vi "SphereSecP(t).vi"(6 "strip (cm)":cluster{"radius":dbl, "h":dbl, "w":dbl}={"radius"=10.0, "h"=5.0, "w"=4.0} {"radius" format="%.2f"; "w" format="%.2f"; "h" format="%.2f"}, 7 "Cluster":T1={"r"=0.0, "d"=0.0, "c (cm/s)"=150000.0, "waveform samp rate s"=1500.0, "In focal Zone?"=FALSE} {"r" format="%.2f"; "d" format="%.2f"; "waveform samp rate s" format="%.2e"; "c (cm/s)" format="%.2f"}, 8 "d (depth of curvature)":dbl format="%.2f", 9 "Drive signal":dbl[](array[numeric])=[-0.5634920634920635, -0.6825396825396826, -0.8015873015873016, -0.9920634920634921, -1.1507936507936507, -1.3888888888888888, -1.992063492063492, -4.2063492063492065, -5.888888888888889, 13.023809523809524, 61.32539682539682, 92.83333333333333, 75.10317460317461, 18.126984126984127, -54.93650793650794, -109.60317460317461, -104.22222222222223, 18.134920634920636, 83.33333333333333, 27.27777777777778, -42.19047619047619, -45.63492063492063, 10.15079365079365, 49.05555555555556, 28.19047619047619, -5.658730158730159, -15.261904761904763, -4.4603174603174605, 7.984126984126984, 10.682539682539682, 5.809523809523809, -0.03968253968253968, -2.515873015873016, -1.4841269841269842, 1.0396825396825398, 2.0555555555555554, 0.9523809523809523, -0.6031746031746031, -1.007936507936508, -0.3968253968253968, 0.14285714285714285] format="%.2f", 10 "edge points":dbl[][](array[numeric]) format="%.2f", 11 "P (cm)":cluster{"x":dbl, "y":dbl, "z":dbl}={"x"=-4.0, "y"=0.0, "z"=4.0} {"x" format="%.2f"; "z" format="%.2f"; "y" format="%.2f"}) -> (2 "Pressure Wave":dbl[](graph), 3 "min time shift":dbl format="%.2f")   [LabVIEW 2022 SP3]
uses:
  <vilib>/Analysis/2dsp.llb/1D Convolution (DBL).vi
  <vilib>/Analysis/baseanly.llb/A x Vector.vi
  <vilib>/Analysis/2dsp.llb/Derivative x(t).vi
  <vilib>/Analysis/NI_AALPro.lvlib
  <vilib>/Analysis/NI_AALBase.lvlib
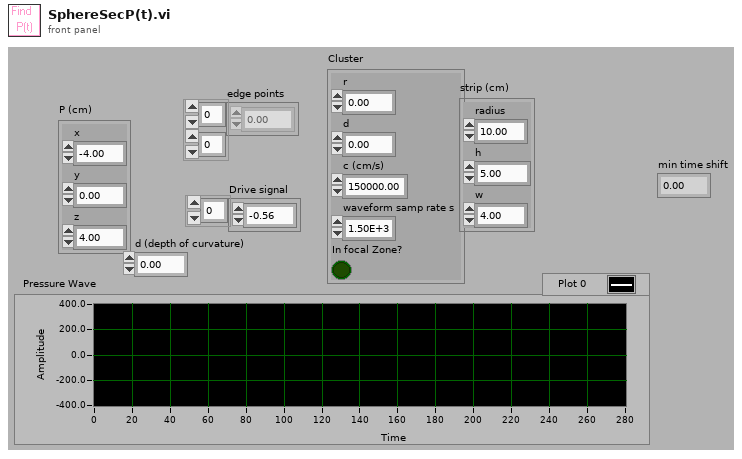
[diagram p1: front panel]
types:
  T1 = cluster{"r":dbl, "d":dbl, "c (cm/s)":dbl, "waveform samp rate s":dbl, "In focal Zone?":bool}
  T2 = cluster{"Number of rings":i32, "sound spd (cm/s)":i32, "z span (cm)":dbl, "z steps":i32, "y span (cm)":dbl, "y steps":i32, "time step (s)":sgl, "z":dbl, "y":dbl, "ref delay":dbl, "freq (MHz)":dbl, "cycles":i32}
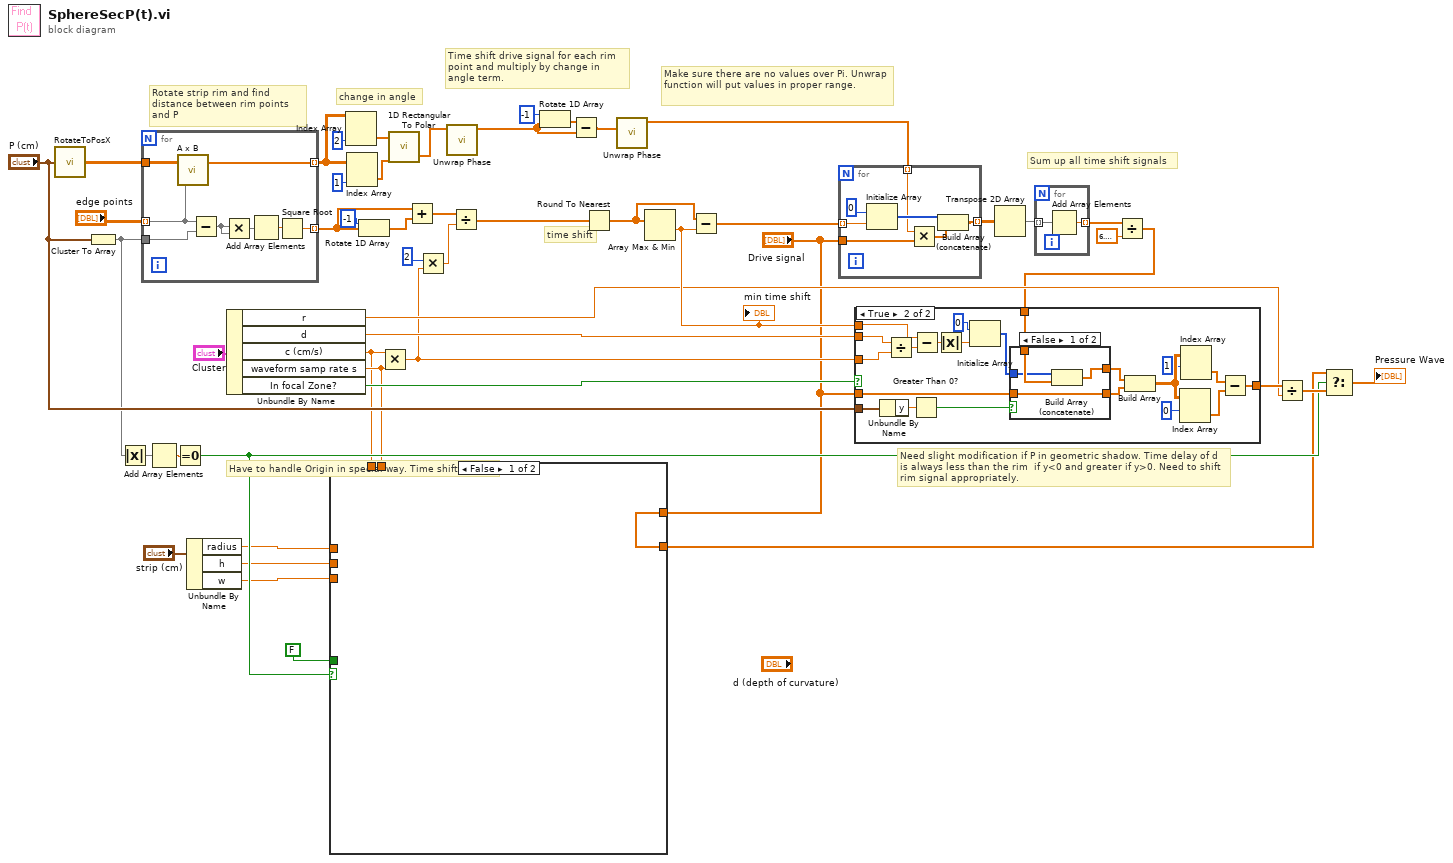
[diagram p0: block diagram]
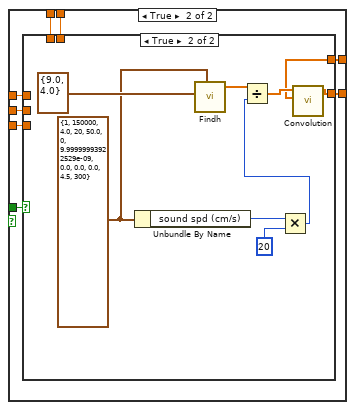
[diagram p2: hidden frame]
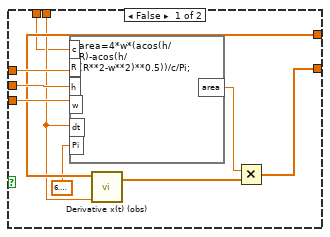
[diagram p3: hidden frame]
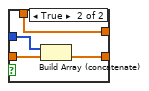
[diagram p5: hidden frame]
diagram:
  # "Have to handle Origin in special way. Time shift is R"
  # "Make sure there are no values over Pi. Unwrap function will put values in proper range."
  # "Need slight modification if P in geometric shadow. Time delay of d is always less than the rim  if y<0 and greater if y>0. Need to shift rim signal appropriately."
  # "Sum up all time shift signals"
  # "Time shift drive signal for each rim point and multiply by change in angle term."
  # "Rotate strip rim and find distance between rim points and P"
  # "time shift"
  # "change in angle"
  n1 = call "RotateToPosX.vi"("P"="P (cm)") -> ("Rotatation Matrix"=w29:dbl[][])
  n2 = Cluster To Array(cluster="P (cm)") -> (array=w25:dbl[])
  n3 = Absolute Value(x=w25) -> (abs(x)=w22:dbl[])
  n4 = for {
    tunnel: "edge points" -> [w57] mode=indexing
    tunnel: w29 -> [w58]
    tunnel: [w51] -> w19 mode=indexing
    tunnel: w25 -> [w56]
    tunnel: [w52] -> w35 mode=indexing
    n5 = call-poly <vilib>:"A x B.vi"("Vector"=w57, "A"=w58) -> ("A x Vector"=w51:dbl[])  [unwired: 1 out]
    n6 = Subtract(x=w57, y=w56) -> (x-y=w55:dbl[])
    n7 = Multiply(x=w55, y=w55) -> (x*y=w54:dbl[])
    n8 = Add Array Elements(numeric array=w54) -> (sum=w53:dbl)
    n9 = Square Root(x=w53) -> (sqrt(x)=w52:dbl)
  }
  n10 = Add Array Elements(numeric array=w22) -> (sum=w24:dbl)
  n11 = Equal To 0?(x=w24) -> (x = 0?=w10:bool)
  n12 = Unbundle By Name("strip (cm)") -> ("radius"=w4:dbl, "h"=w6:dbl, "w"=w5:dbl)
  n13 = Unbundle By Name("Cluster") -> ("r"=w32:dbl, "d"=w39:dbl, "c (cm/s)"=w2:dbl, "waveform samp rate s"=w3:dbl, "In focal Zone?"=w16:bool)
  n14 = case shown="False" w10 {
    tunnel: "Drive signal" -> [w59 w67]
    tunnel: [w59 w66] -> w1
    tunnel: FALSE -> [_ w65]
    tunnel: w6 -> [_ w64]
    tunnel: w5 -> [_ w63]
    tunnel: w4 -> [_ w62]
    tunnel: w3 -> [_ w61]
    tunnel: w2 -> [_ w60]
    frame False {
    }
    frame True {
      n15 = case shown="True" w65 {
        tunnel: w67 -> [w74 w82]
        tunnel: [w69 w81] -> w66
        tunnel: w64 -> [w77 _]
        tunnel: w63 -> [w76 _]
        tunnel: w62 -> [w75 _]
        tunnel: w61 -> [w73 _]
        tunnel: w60 -> [w70 _]
        frame False {
          n16 = formula code="area=4*w*(acos(h/R)-acos(h/(R**2-w**2)**0.5))/c/Pi;"("R"=w75, "w"=w76, "h"=w77, "dt"=w73, "c"=w70, "Pi"=6.283185307179586) -> ("area"=w71:dbl)
          n17 = call <vilib>:"Derivative x(t) (obs).vi"("dt"=w73, "X"=w74) -> ("dX/dt"=w72:dbl[])  [unwired: 2 in, 1 out]
          n18 = Multiply(x=w71, y=w72) -> (x*y=w69:dbl[])
        }
        frame True {
          w85 = T2 {"Number of rings"=1, "sound spd (cm/s)"=150000, "z span (cm)"=4.0, "z steps"=20, "y span (cm)"=50.0, "y steps"=0, "time step (s)"=1e-08, "z"=0.0, "y"=0.0, "ref delay"=0.0, "freq (MHz)"=4.5, "cycles"=300} ("Variables in")
          n19 = Unbundle By Name(w85) -> ("sound spd (cm/s)"=w80:i32)
          n20 = call "Findh.vi"("Trans Geometry"=cluster{"Radius":dbl, "a":dbl} {"Radius"=9.0, "a"=4.0}, "Variables in"=w85) -> ("h(r,t)"=w84:dbl[])  [unwired: 1 in, 4 out]
          n21 = Multiply(x=w80, y=20) -> (x*y=w78:i32)
          n22 = Divide(x=w84, y=w78) -> (x/y=w83:dbl[])
          n23 = call-poly <vilib>:"Convolution.vi"("Y"=w82, "X"=w83) -> ("X * Y"=w81:dbl[])  [unwired: 1 in, 8 out]
        }
      }
    }
  }
  n24 = Index Array(array=w19, index (col)=2) -> (element=w48:dbl[])  [unwired: 1 in]
  n25 = Index Array(array=w19, index (col)=1) -> (element=w26:dbl[])  [unwired: 1 in]
  n26 = Rotate 1D Array(1:w35, 2:-1) -> (0:w34:dbl[])
  n27 = Multiply(x=w2, y=w3) -> (x*y=w30:dbl)
  n28 = call <vilib>:"1D Rectangular To Polar.vi"("X"=w48, "Y"=w26) -> ("Phase"=w14:dbl[])  [unwired: 2 out]
  n29 = Add(x=w35, y=w34) -> (x+y=w45:dbl[])
  n30 = Multiply(x=2, y=w30) -> (x*y=w43:dbl)
  n31 = call <vilib>:"Unwrap Phase.vi"("Phase"=w14) -> ("Unwrapped Phase"=w13:dbl[])  [unwired: 1 in, 9 out]
  n32 = Divide(x=w45, y=w43) -> (x/y=w31:dbl[])
  n33 = Rotate 1D Array(1:w13, 2:-1) -> (0:w15:dbl[])
  n34 = Subtract(x=w15, y=w13) -> (x-y=w12:dbl[])
  n35 = Round To Nearest(number=w31) -> (nearest integer value=w42:dbl[])
  n36 = call <vilib>:"Unwrap Phase.vi"("Phase"=w12) -> ("Unwrapped Phase"=w11:dbl[])  [unwired: 1 in, 9 out]
  n37 = Array Max & Min(array=w42) -> (min value=w38:dbl)  [unwired: 3 out]
  "min time shift" <- w38
  n38 = Subtract(x=w42, y=w38) -> (x-y=w21:dbl[])
  n39 = for {
    tunnel: w21 -> [w93] mode=indexing
    tunnel: "Drive signal" -> [w90]
    tunnel: [w87] -> w17 mode=indexing
    tunnel: w11 -> [w88] mode=indexing
    n40 = Initialize Array(0, w93) -> (w91:i32[])
    n41 = Multiply(x=w88, y=w90) -> (x*y=w89:dbl[])
    n42 = Build Array (concatenate)(w91, w89) -> (w87:dbl[])
  }
  n43 = Transpose 2D Array(2D array=w17) -> (transposed array=w41:dbl[][])
  n44 = for {
    tunnel: w41 -> [w95] mode=indexing
    tunnel: [w94] -> w37 mode=indexing
    n45 = Add Array Elements(numeric array=w95) -> (sum=w94:dbl)
  }
  n46 = Divide(x=w37, y=6.283185307179586) -> (x/y=w20:dbl[])
  n47 = case shown="True" w16 {
    tunnel: w39 -> [_ w117]
    tunnel: w20 -> [w96 w99]
    tunnel: [w96 w115] -> w33
    tunnel: "Drive signal" -> [_ w104]
    tunnel: w38 -> [_ w106]
    tunnel: "P (cm)" -> [_ w108]
    tunnel: w30 -> [_ w105]
    frame False {
      # "No mods if P not in geometric shadow"
    }
    frame True {
      n48 = Unbundle By Name(w108) -> ("y"=w107:dbl)
      n49 = Divide(x=w117, y=w105) -> (x/y=w109:dbl)
      n50 = Greater Than 0?(x=w107) -> (x > 0?=w102:bool)
      n51 = Subtract(x=w106, y=w109) -> (x-y=w116:dbl)
      n52 = Absolute Value(x=w116) -> (abs(x)=w100:dbl)
      n53 = Initialize Array(0, w100) -> (w98:i32[])
      n54 = case shown="False" w102 {
        tunnel: [w121 w122] -> w97
        tunnel: [w120 w123] -> w103
        tunnel: w104 -> [w120 w124]
        tunnel: w99 -> [w119 w122]
        tunnel: w98 -> [w118 w125]
        frame False {
          n55 = Build Array (concatenate)(w118, w119) -> (w121:dbl[])
        }
        frame True {
          n56 = Build Array (concatenate)(w125, w124) -> (w123:dbl[])
        }
      }
      n57 = Build Array(w97, w103) -> (w114:dbl[][])
      n58 = Index Array(array=w114, index (row)=0) -> (element=w111:dbl[])  [unwired: 1 in]
      n59 = Index Array(array=w114, index (row)=1) -> (element=w110:dbl[])  [unwired: 1 in]
      n60 = Subtract(x=w110, y=w111) -> (x-y=w115:dbl[])
    }
  }
  n61 = Divide(x=w33, y=w32) -> (x/y=w23:dbl[])
  n62 = Select(t=w1, s=w10, f=w23) -> (s? t:f=→"Pressure Wave":dbl[])
